vi "XYZ stage handler_MD.vi"   [LabVIEW 2012]
uses:
  <vilib>/Analysis/coordinate.llb/Euler Rotation Order.ctl
  GFG/GFGfpRefGet.vi
  GFG/GFGbooleanGet.vi
  GFG/GFGnumericGet.vi
  <vilib>/Analysis/coordinate.llb/3D Cartesian Coordinate Rotation (Euler) (Scalar).vi
  GFG/GFG library.lvlib
  <vilib>/Utility/VariantDataType/Type.ctl
  <vilib>/Utility/VariantDataType/VariantType.lvlib
  <vilib>/Analysis/NI_AALPro.lvlib
types:
  T1 = enum16{"none", "quit", "Press", "Long Press", "Long Press finished", "Short Press finished"}
  T2 = cluster{"WaveformChartRef":refnum<vi>, "DigitalRef":refnum<vi>, "ArrayRef":refnum<vi>, "TabControlRef":refnum<vi>, "EnumRef":refnum<vi>, "RingRef":refnum<vi>, "BooleanRef":refnum<vi>, "KnobRef":refnum<vi>, "SlideRef":refnum<vi>, "PathRef":refnum<vi>, "StringRef":refnum<vi>, "ComboBox":refnum<vi>, "WaveformGraphRef":refnum<vi>}
  T3 = cluster{"moveXabs":dbl, "moveYabs":dbl, "moveZabs":dbl}
  T4 = typedef "NI_AALPro.lvlib/Euler Rotation Order.ctl" = u16
  T5 = cluster{"Numeric":dbl, "Numeric":dbl, "Numeric":dbl}
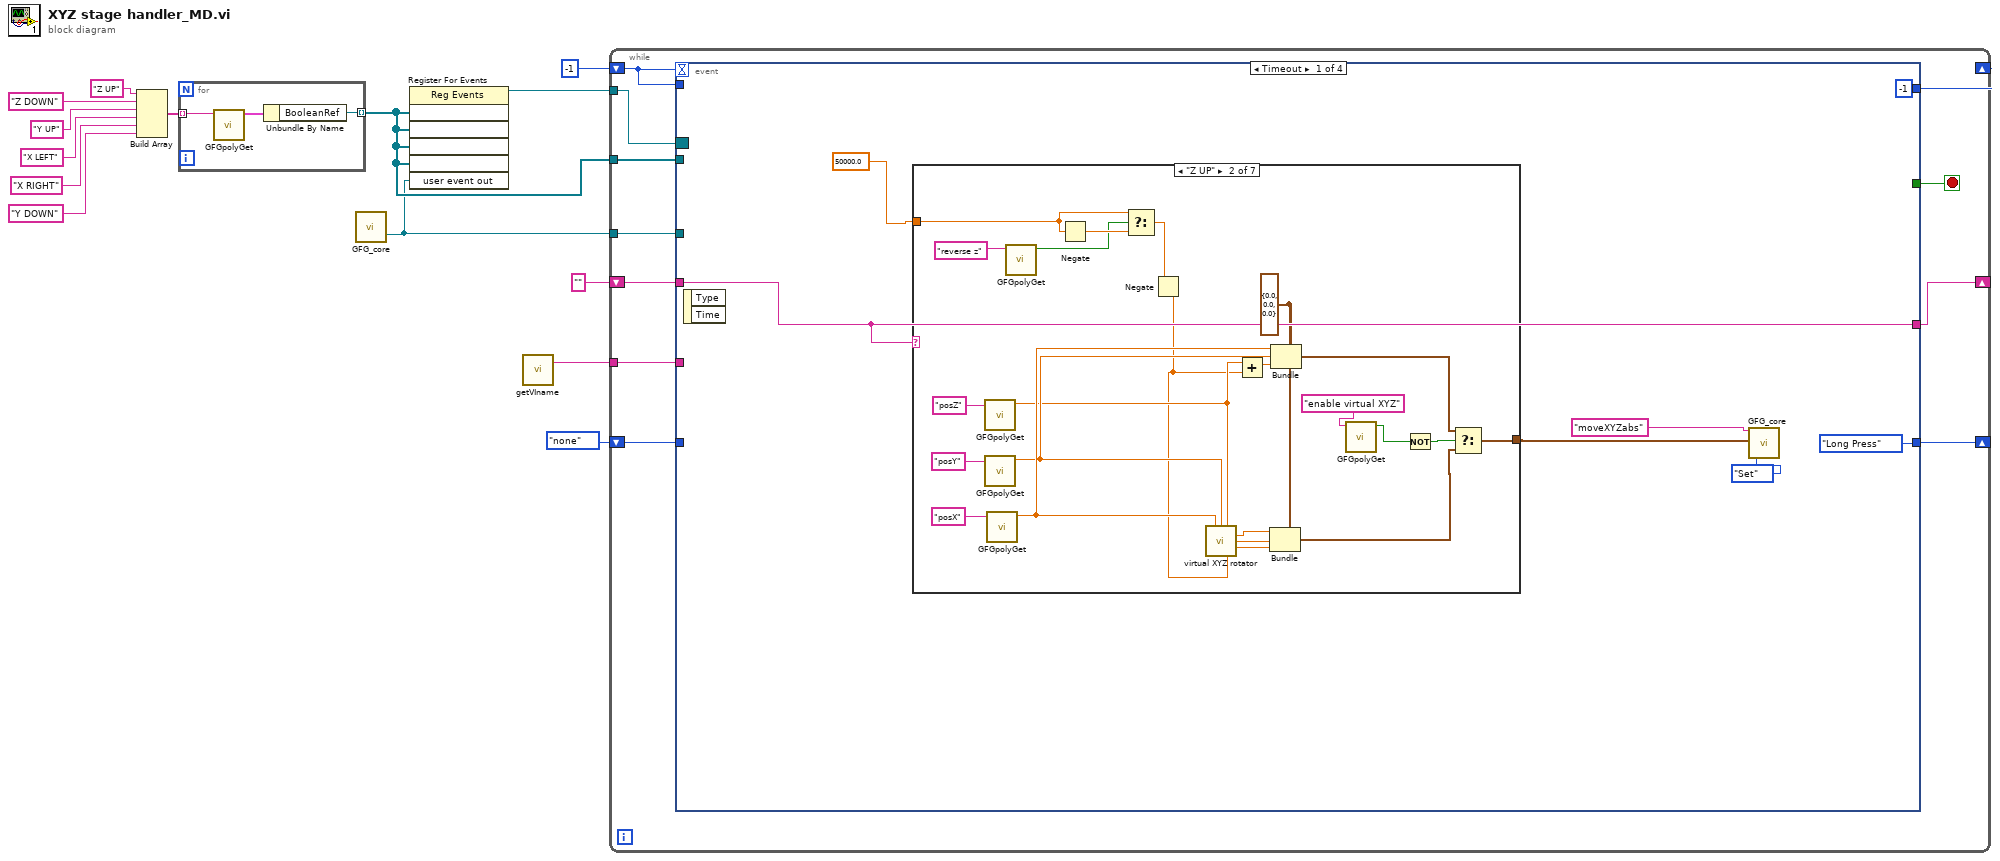
[diagram p0: block diagram]
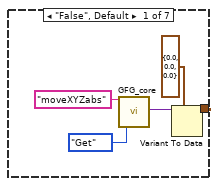
[diagram p2: hidden frame]
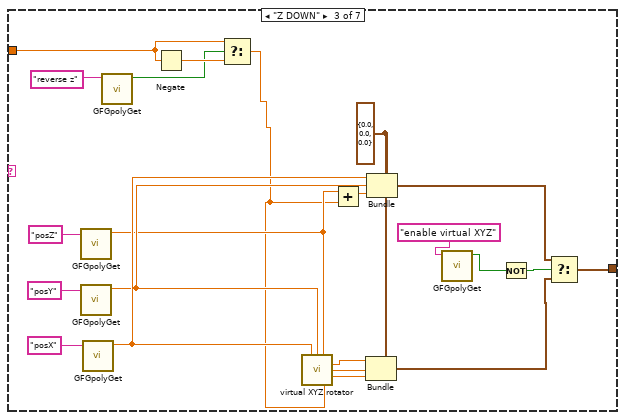
[diagram p3: hidden frame]
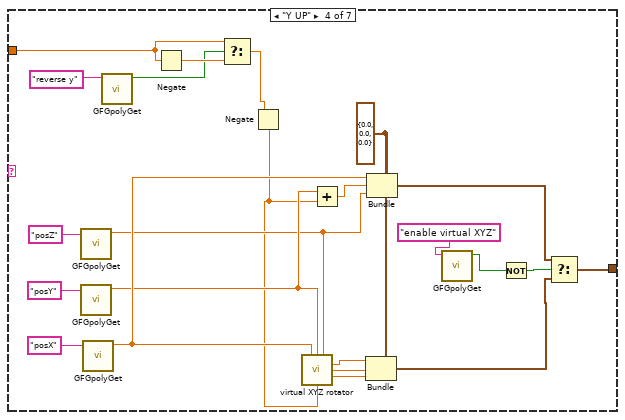
[diagram p4: hidden frame]
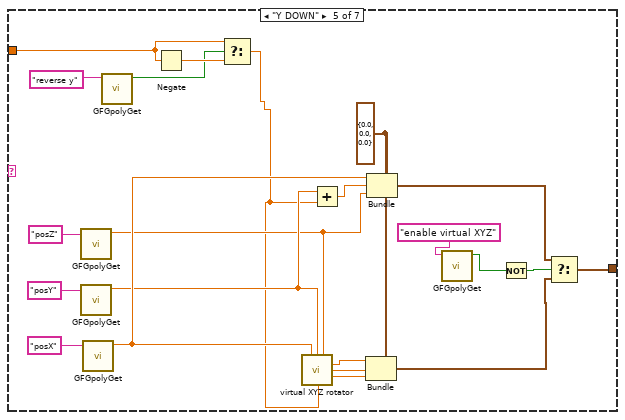
[diagram p5: hidden frame]
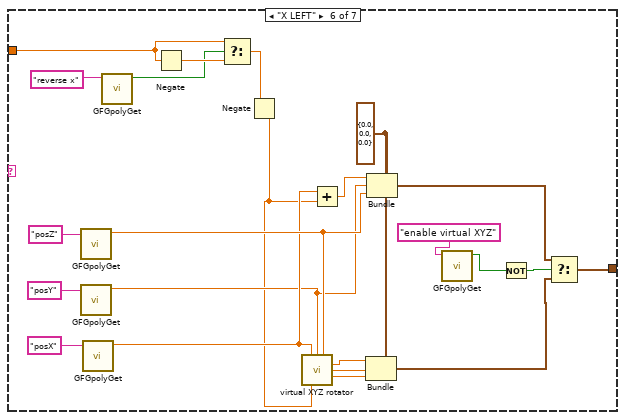
[diagram p6: hidden frame]
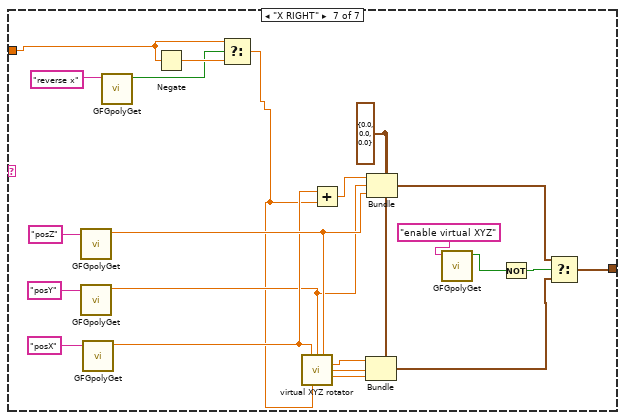
[diagram p7: hidden frame]
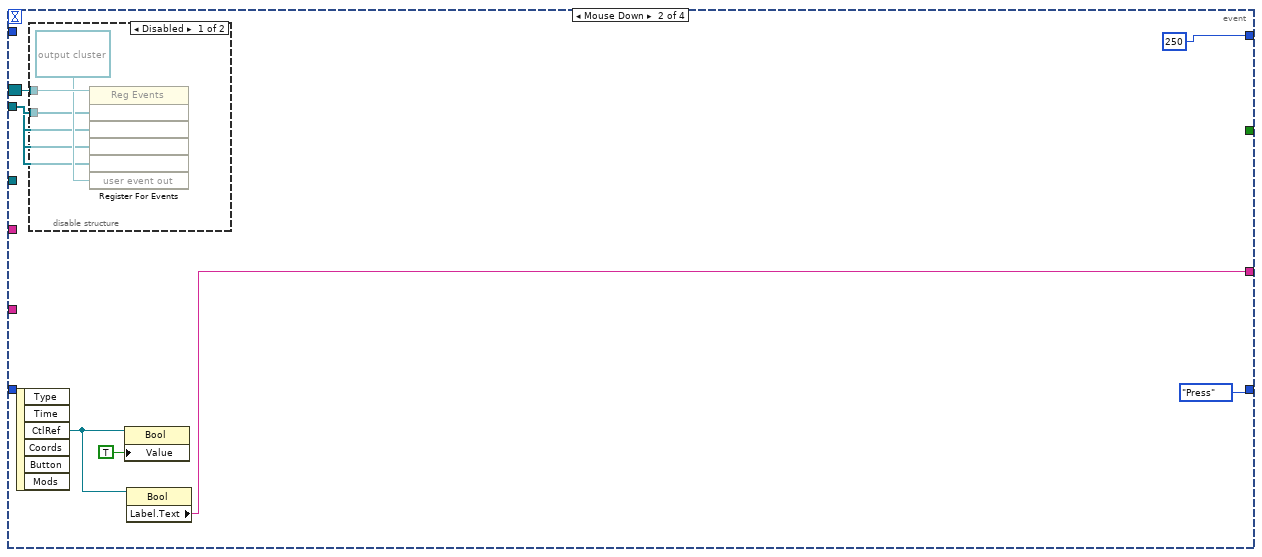
[diagram p8: hidden frame]
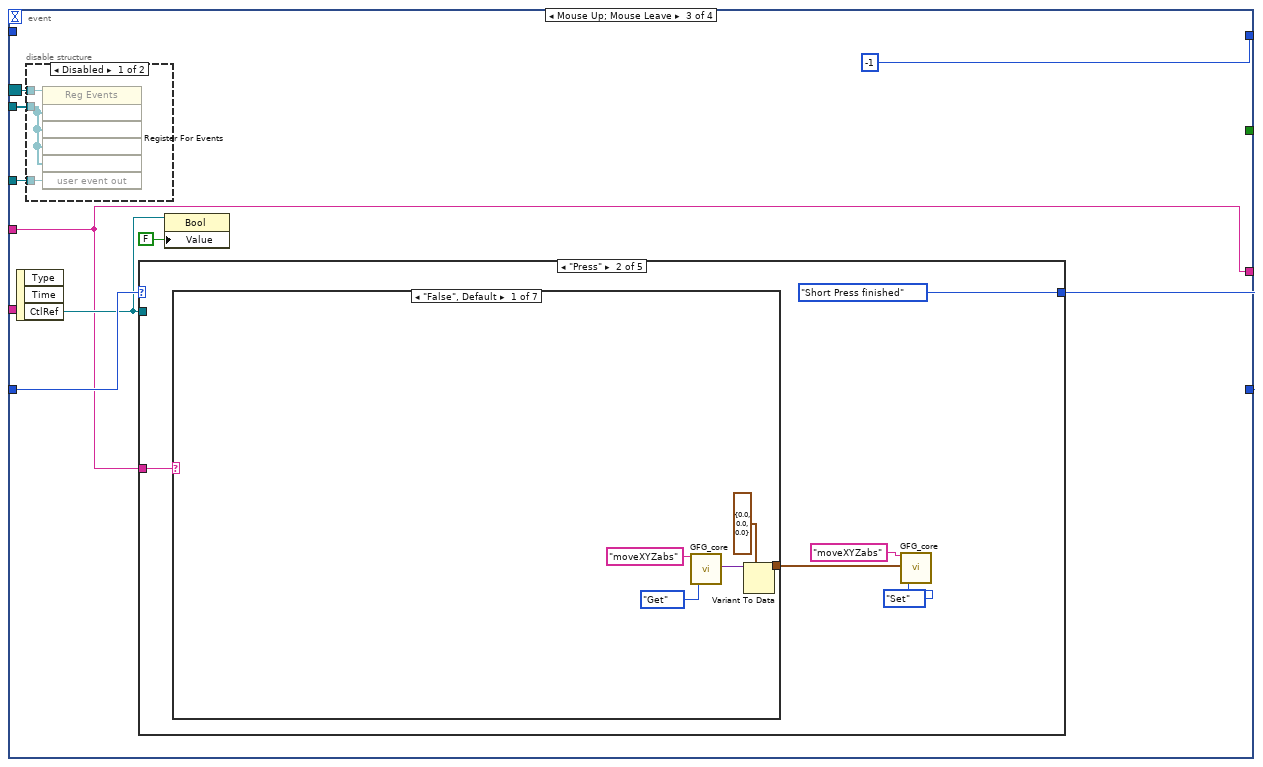
[diagram p10: hidden frame]
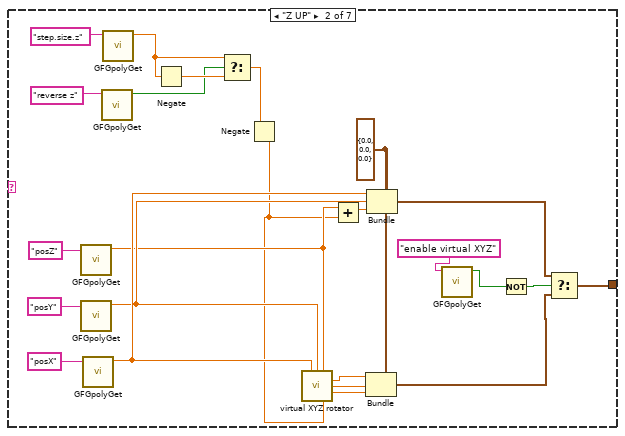
[diagram p13: hidden frame]
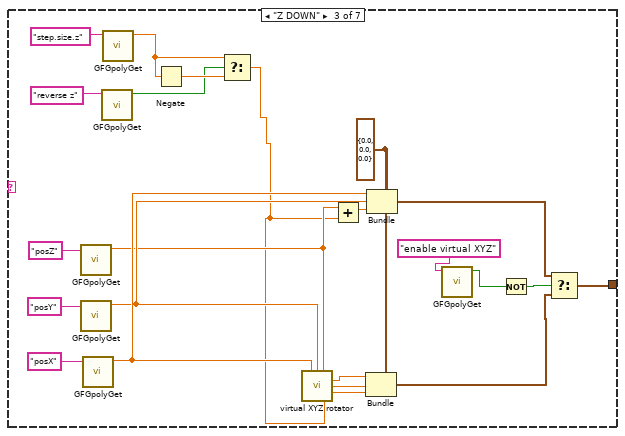
[diagram p14: hidden frame]
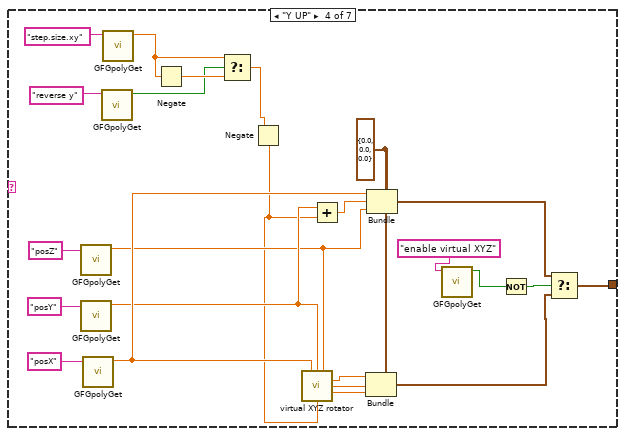
[diagram p15: hidden frame]
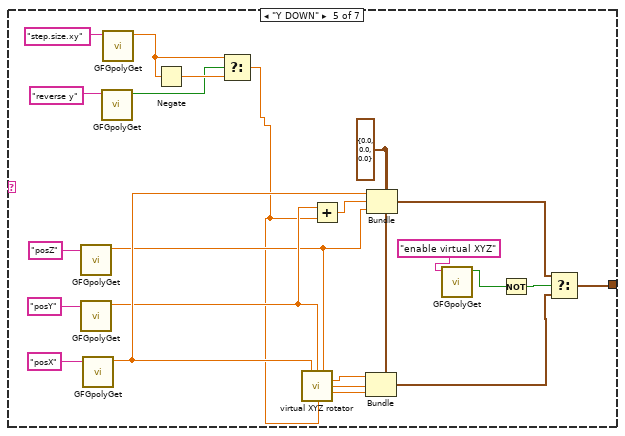
[diagram p16: hidden frame]
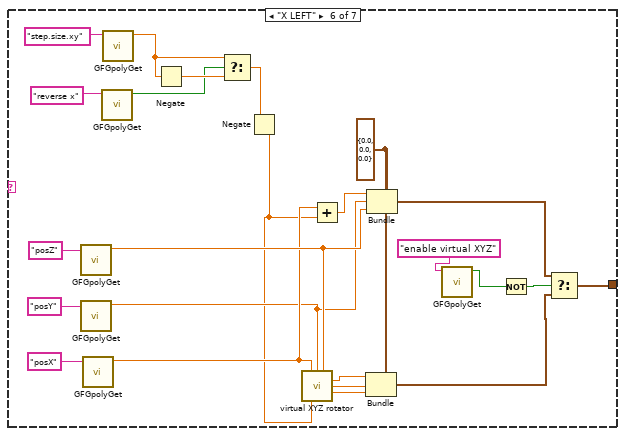
[diagram p17: hidden frame]
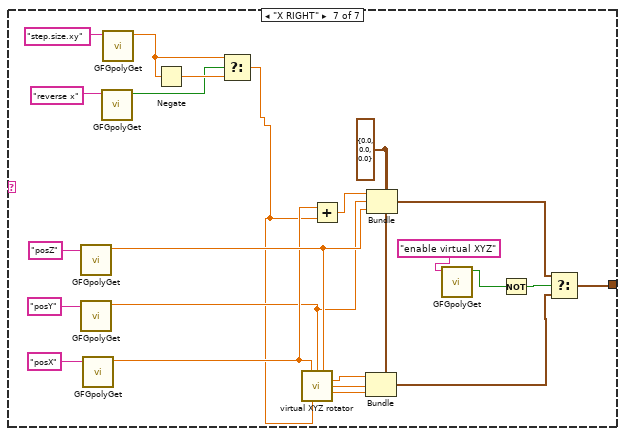
[diagram p18: hidden frame]
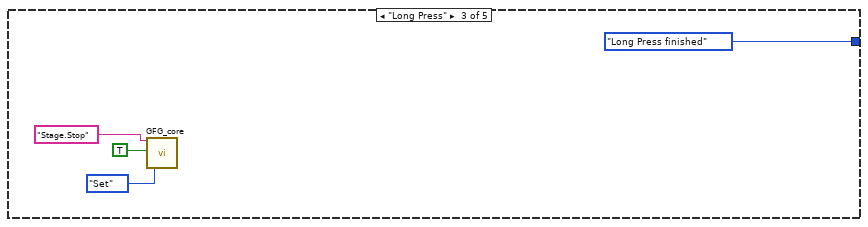
[diagram p19: hidden frame]
diagram:
  n1 = Build Array("Z UP" ("Variable Name in"), "Z DOWN" ("Variable Name in"), "Y UP" ("Variable Name in"), "X LEFT" ("Variable Name in"), "X RIGHT" ("Variable Name in"), "Y DOWN" ("Variable Name in")) -> (w11:string[])
  n2 = for {
    tunnel: w11 -> [w16] mode=indexing
    tunnel: [w15] -> w3 mode=indexing
    n3 = call-poly "GFGpolyGet.vi"("Variable Name in"=w16) -> ("output cluster"=w17:T2)  [unwired: 9 in, 1 out]
    n4 = Unbundle By Name(w17) -> ("BooleanRef"=w15:refnum<vi>)
  }
  n5 = call "GFG_core.vi"() -> ("user event out"=w2:refnum<user-event>)  [unwired: 13 in, 6 out]
  n6 = register-events(w3, w3, w3, w3, w2) -> (reference out=w4:refnum<event-registration>)  [unwired: 2 in, 1 out]
  n7 = call "getVIname.vi"() -> ("VI name"=w1:string)  [unwired: 19 in]
  n8 = while {
    shift-right: [w26] -> _
    shift-left: -1 -> [w27]
    shift-right: [w24] -> _
    shift-left: T1."none" ("Enum") -> [w25]
    shift-right: [w23] -> _
    shift-left: "" ("Label.Text") -> [w22]
    tunnel: w3 -> [w21]
    tunnel: w2 -> [w20]
    tunnel: w4 -> [w19]
    tunnel: w1 -> [w18]
    stop <- w28 stop-if-true
    n9 = event shown="[0] Timeout" {
      selector: w19 -> [_ w179 w188 _]
      dyn-events: _ -> [_ _ _ _]
      timeout: w27 -> [_ _ _ _]
      tunnel: [_ _ _ w361] -> w28
      tunnel: w27 -> [_ _ _ w359]
      tunnel: [-1 250 -1 w359] -> w26
      tunnel: w25 -> [_ _ w193 w360]
      tunnel: [T1."Long Press" ("Enum") T1."Press" ("Enum") w192 w360] -> w24
      tunnel: [w33 w180 w186 w356] -> w23
      tunnel: w22 -> [w33 _ w186 w356]
      tunnel: w21 -> [_ w176 w187 _]
      tunnel: w20 -> [_ _ w189 _]
      tunnel: w18 -> [_ _ _ w357]
      event Timeout {
        n10 = event-data() -> ()  [unwired: 1 in, 2 out]
        n11 = case shown="\"Z UP\"" w33 {
          tunnel: [w36 w46 w68 w94 w116 w140 w162] -> w29
          tunnel: 50000.0 ("-x") -> [_ w41 w64 w86 w109 w131 w154]
          frame "False", Default {
            n12 = call "GFG_core.vi"("Variable Name in"="moveXYZabs", "Action"=enum16{"Init", "Set", "Get"}."Get") -> ("Variant Out"=w38:variant)  [unwired: 11 in, 6 out]
            n13 = Variant To Data(type=T3 {"moveXabs"=0.0, "moveYabs"=0.0, "moveZabs"=0.0} ("output cluster"), Variant=w38) -> (data=w36:T3)  [unwired: 1 in, 1 out]
          }
          frame "Z UP" {
            w49 = T3 {"moveXabs"=0.0, "moveYabs"=0.0, "moveZabs"=0.0} ("output cluster")
            n14 = call-poly "GFGpolyGet.vi"("Variable Name in"="posZ") -> ("Numeric"=w53:dbl)  [unwired: 9 in, 1 out]
            n15 = call-poly "GFGpolyGet.vi"("Variable Name in"="posY") -> ("Numeric"=w54:dbl)  [unwired: 9 in, 1 out]
            n16 = call-poly "GFGpolyGet.vi"("Variable Name in"="posX") -> ("Numeric"=w55:dbl)  [unwired: 9 in, 1 out]
            n17 = call-poly "GFGpolyGet.vi"("Variable Name in"="reverse z") -> ("Boolean"=w61:bool)  [unwired: 10 in]
            n18 = Negate(x=w41) -> (-x=w62:dbl)
            n19 = Select(t=w41, s=w61, f=w62) -> (s? t:f=w43:dbl)
            n20 = Negate(x=w43) -> (-x=w42:dbl)
            n21 = call "virtual XYZ rotator.vi"("current pos X"=w55, "current pos Y"=w54, "current pos Z"=w53, "virtual Z relative"=w42) -> ("new pos X"=w52:dbl, "new pos Y"=w51:dbl, "new pos Z"=w50:dbl)  [unwired: 9 in]
            n22 = Add(x=w53, y=w42) -> (x+y=w57:dbl)
            n23 = Bundle(cluster=w49, "moveXabs"=w52, "moveYabs"=w51, "moveZabs"=w50) -> (w47:T3)
            n24 = Bundle(cluster=w49, "moveXabs"=w55, "moveYabs"=w54, "moveZabs"=w57) -> (w48:T3)
            n25 = call-poly "GFGpolyGet.vi"("Variable Name in"="enable virtual XYZ") -> ("Boolean"=w45:bool)  [unwired: 10 in]
            n26 = Not(x=w45) -> (.not. x?=w44:bool)
            n27 = Select(t=w48, s=w44, f=w47) -> (s? t:f=w46:T3)
          }
          frame "Z DOWN" {
            w71 = T3 {"moveXabs"=0.0, "moveYabs"=0.0, "moveZabs"=0.0} ("output cluster")
            n28 = call-poly "GFGpolyGet.vi"("Variable Name in"="posZ") -> ("Numeric"=w75:dbl)  [unwired: 9 in, 1 out]
            n29 = call-poly "GFGpolyGet.vi"("Variable Name in"="posY") -> ("Numeric"=w76:dbl)  [unwired: 9 in, 1 out]
            n30 = call-poly "GFGpolyGet.vi"("Variable Name in"="posX") -> ("Numeric"=w77:dbl)  [unwired: 9 in, 1 out]
            n31 = call-poly "GFGpolyGet.vi"("Variable Name in"="reverse z") -> ("Boolean"=w83:bool)  [unwired: 10 in]
            n32 = Negate(x=w64) -> (-x=w84:dbl)
            n33 = Select(t=w64, s=w83, f=w84) -> (s? t:f=w65:dbl)
            n34 = call "virtual XYZ rotator.vi"("current pos X"=w77, "current pos Y"=w76, "current pos Z"=w75, "virtual Z relative"=w65) -> ("new pos X"=w74:dbl, "new pos Y"=w73:dbl, "new pos Z"=w72:dbl)  [unwired: 9 in]
            n35 = Add(x=w75, y=w65) -> (x+y=w79:dbl)
            n36 = Bundle(cluster=w71, "moveXabs"=w74, "moveYabs"=w73, "moveZabs"=w72) -> (w69:T3)
            n37 = Bundle(cluster=w71, "moveXabs"=w77, "moveYabs"=w76, "moveZabs"=w79) -> (w70:T3)
            n38 = call-poly "GFGpolyGet.vi"("Variable Name in"="enable virtual XYZ") -> ("Boolean"=w67:bool)  [unwired: 10 in]
            n39 = Not(x=w67) -> (.not. x?=w66:bool)
            n40 = Select(t=w70, s=w66, f=w69) -> (s? t:f=w68:T3)
          }
          frame "Y UP" {
            w97 = T3 {"moveXabs"=0.0, "moveYabs"=0.0, "moveZabs"=0.0} ("output cluster")
            n41 = call-poly "GFGpolyGet.vi"("Variable Name in"="posZ") -> ("Numeric"=w88:dbl)  [unwired: 9 in, 1 out]
            n42 = call-poly "GFGpolyGet.vi"("Variable Name in"="posY") -> ("Numeric"=w90:dbl)  [unwired: 9 in, 1 out]
            n43 = call-poly "GFGpolyGet.vi"("Variable Name in"="posX") -> ("Numeric"=w101:dbl)  [unwired: 9 in, 1 out]
            n44 = call-poly "GFGpolyGet.vi"("Variable Name in"="reverse y") -> ("Boolean"=w106:bool)  [unwired: 10 in]
            n45 = Negate(x=w86) -> (-x=w107:dbl)
            n46 = Select(t=w86, s=w106, f=w107) -> (s? t:f=w91:dbl)
            n47 = Negate(x=w91) -> (-x=w87:dbl)
            n48 = call "virtual XYZ rotator.vi"("current pos X"=w101, "current pos Y"=w90, "current pos Z"=w88, "virtual Y relative"=w87) -> ("new pos X"=w100:dbl, "new pos Y"=w99:dbl, "new pos Z"=w98:dbl)  [unwired: 9 in]
            n49 = Add(x=w90, y=w87) -> (x+y=w89:dbl)
            n50 = Bundle(cluster=w97, "moveXabs"=w100, "moveYabs"=w99, "moveZabs"=w98) -> (w95:T3)
            n51 = Bundle(cluster=w97, "moveXabs"=w101, "moveYabs"=w89, "moveZabs"=w88) -> (w96:T3)
            n52 = call-poly "GFGpolyGet.vi"("Variable Name in"="enable virtual XYZ") -> ("Boolean"=w93:bool)  [unwired: 10 in]
            n53 = Not(x=w93) -> (.not. x?=w92:bool)
            n54 = Select(t=w96, s=w92, f=w95) -> (s? t:f=w94:T3)
          }
          frame "Y DOWN" {
            w119 = T3 {"moveXabs"=0.0, "moveYabs"=0.0, "moveZabs"=0.0} ("output cluster")
            n55 = call-poly "GFGpolyGet.vi"("Variable Name in"="posZ") -> ("Numeric"=w111:dbl)  [unwired: 9 in, 1 out]
            n56 = call-poly "GFGpolyGet.vi"("Variable Name in"="posY") -> ("Numeric"=w113:dbl)  [unwired: 9 in, 1 out]
            n57 = call-poly "GFGpolyGet.vi"("Variable Name in"="posX") -> ("Numeric"=w123:dbl)  [unwired: 9 in, 1 out]
            n58 = call-poly "GFGpolyGet.vi"("Variable Name in"="reverse y") -> ("Boolean"=w128:bool)  [unwired: 10 in]
            n59 = Negate(x=w109) -> (-x=w129:dbl)
            n60 = Select(t=w109, s=w128, f=w129) -> (s? t:f=w110:dbl)
            n61 = call "virtual XYZ rotator.vi"("current pos X"=w123, "current pos Y"=w113, "current pos Z"=w111, "virtual Y relative"=w110) -> ("new pos X"=w122:dbl, "new pos Y"=w121:dbl, "new pos Z"=w120:dbl)  [unwired: 9 in]
            n62 = Add(x=w113, y=w110) -> (x+y=w112:dbl)
            n63 = Bundle(cluster=w119, "moveXabs"=w122, "moveYabs"=w121, "moveZabs"=w120) -> (w117:T3)
            n64 = Bundle(cluster=w119, "moveXabs"=w123, "moveYabs"=w112, "moveZabs"=w111) -> (w118:T3)
            n65 = call-poly "GFGpolyGet.vi"("Variable Name in"="enable virtual XYZ") -> ("Boolean"=w115:bool)  [unwired: 10 in]
            n66 = Not(x=w115) -> (.not. x?=w114:bool)
            n67 = Select(t=w118, s=w114, f=w117) -> (s? t:f=w116:T3)
          }
          frame "X LEFT" {
            w143 = T3 {"moveXabs"=0.0, "moveYabs"=0.0, "moveZabs"=0.0} ("output cluster")
            n68 = call-poly "GFGpolyGet.vi"("Variable Name in"="posZ") -> ("Numeric"=w137:dbl)  [unwired: 9 in, 1 out]
            n69 = call-poly "GFGpolyGet.vi"("Variable Name in"="posY") -> ("Numeric"=w134:dbl)  [unwired: 9 in, 1 out]
            n70 = call-poly "GFGpolyGet.vi"("Variable Name in"="posX") -> ("Numeric"=w136:dbl)  [unwired: 9 in, 1 out]
            n71 = call-poly "GFGpolyGet.vi"("Variable Name in"="reverse x") -> ("Boolean"=w151:bool)  [unwired: 10 in]
            n72 = Negate(x=w131) -> (-x=w152:dbl)
            n73 = Select(t=w131, s=w151, f=w152) -> (s? t:f=w133:dbl)
            n74 = Negate(x=w133) -> (-x=w132:dbl)
            n75 = call "virtual XYZ rotator.vi"("current pos X"=w136, "current pos Y"=w134, "current pos Z"=w137, "virtual X relative"=w132) -> ("new pos X"=w146:dbl, "new pos Y"=w145:dbl, "new pos Z"=w144:dbl)  [unwired: 9 in]
            n76 = Add(x=w136, y=w132) -> (x+y=w135:dbl)
            n77 = Bundle(cluster=w143, "moveXabs"=w146, "moveYabs"=w145, "moveZabs"=w144) -> (w141:T3)
            n78 = Bundle(cluster=w143, "moveXabs"=w135, "moveYabs"=w134, "moveZabs"=w137) -> (w142:T3)
            n79 = call-poly "GFGpolyGet.vi"("Variable Name in"="enable virtual XYZ") -> ("Boolean"=w139:bool)  [unwired: 10 in]
            n80 = Not(x=w139) -> (.not. x?=w138:bool)
            n81 = Select(t=w142, s=w138, f=w141) -> (s? t:f=w140:T3)
          }
          frame "X RIGHT" {
            w165 = T3 {"moveXabs"=0.0, "moveYabs"=0.0, "moveZabs"=0.0} ("output cluster")
            n82 = call-poly "GFGpolyGet.vi"("Variable Name in"="posZ") -> ("Numeric"=w159:dbl)  [unwired: 9 in, 1 out]
            n83 = call-poly "GFGpolyGet.vi"("Variable Name in"="posY") -> ("Numeric"=w156:dbl)  [unwired: 9 in, 1 out]
            n84 = call-poly "GFGpolyGet.vi"("Variable Name in"="posX") -> ("Numeric"=w158:dbl)  [unwired: 9 in, 1 out]
            n85 = call-poly "GFGpolyGet.vi"("Variable Name in"="reverse x") -> ("Boolean"=w173:bool)  [unwired: 10 in]
            n86 = Negate(x=w154) -> (-x=w174:dbl)
            n87 = Select(t=w154, s=w173, f=w174) -> (s? t:f=w155:dbl)
            n88 = call "virtual XYZ rotator.vi"("current pos X"=w158, "current pos Y"=w156, "current pos Z"=w159, "virtual X relative"=w155) -> ("new pos X"=w168:dbl, "new pos Y"=w167:dbl, "new pos Z"=w166:dbl)  [unwired: 9 in]
            n89 = Add(x=w158, y=w155) -> (x+y=w157:dbl)
            n90 = Bundle(cluster=w165, "moveXabs"=w168, "moveYabs"=w167, "moveZabs"=w166) -> (w163:T3)
            n91 = Bundle(cluster=w165, "moveXabs"=w157, "moveYabs"=w156, "moveZabs"=w159) -> (w164:T3)
            n92 = call-poly "GFGpolyGet.vi"("Variable Name in"="enable virtual XYZ") -> ("Boolean"=w161:bool)  [unwired: 10 in]
            n93 = Not(x=w161) -> (.not. x?=w160:bool)
            n94 = Select(t=w164, s=w160, f=w163) -> (s? t:f=w162:T3)
          }
        }
        n95 = call "GFG_core.vi"("Variable Name in"="moveXYZabs", "Variant in"=w29, "Action"=enum16{"Init", "Set", "Get"}."Set") -> ()  [unwired: 10 in, 7 out]
      }
      event Mouse Down {
        n96 = event-data() -> ("CtlRef"=w178:refnum<vi>)  [unwired: 1 in, 5 out]
        n97 = disable-structure shown="Disabled" {
          disable-tunnel: w179 -> [w185 _]
          disable-tunnel: w176 -> [w183 _]
          frame Disabled {
            n98 = register-events(reference=w185, w183, w183, w183, w183, refnum<user-event> refnum ("event source")) -> ()  [unwired: 1 in, 2 out]
          }
          frame Enabled {
          }
        }
        n99 = property class="Bool"(reference=w178, "Value"=TRUE) -> ()  [unwired: 1 in, 2 out]
        n100 = property class="Bool"(reference=w178) -> ("Label.Text"=w180:string)  [unwired: 1 in, 2 out]
      }
      event Mouse Up; Mouse Leave {
        n101 = event-data() -> ("CtlRef"=w191:refnum<vi>)  [unwired: 1 in, 2 out]
        n102 = disable-structure shown="Disabled" {
          disable-tunnel: w189 -> [w197 _]
          disable-tunnel: w188 -> [w196 _]
          disable-tunnel: w187 -> [w195 _]
          frame Disabled {
            n103 = register-events(reference=w196, w195, w195, w195, w195, w197) -> ()  [unwired: 1 in, 2 out]
          }
          frame Enabled {
          }
        }
        n104 = case shown="\"Press\"" w193 {
          selector: w193 -> [w198 _ _ w354 w355]
          tunnel: [w198 T1."Short Press finished" ("Enum") T1."Long Press finished" ("Enum") w354 w355] -> w192
          tunnel: w191 -> [_ _ _ _ _]
          tunnel: w186 -> [_ w202 _ _ _]
          frame "none", Default {
          }
          frame "Press" {
            n105 = case shown="\"False\", Default" w202 {
              tunnel: [w204 w213 w236 w263 w286 w311 w334] -> w199
              frame "False", Default {
                n106 = call "GFG_core.vi"("Variable Name in"="moveXYZabs", "Action"=enum16{"Init", "Set", "Get"}."Get") -> ("Variant Out"=w206:variant)  [unwired: 11 in, 6 out]
                n107 = Variant To Data(type=T3 {"moveXabs"=0.0, "moveYabs"=0.0, "moveZabs"=0.0} ("output cluster"), Variant=w206) -> (data=w204:T3)  [unwired: 1 in, 1 out]
              }
              frame "Z UP" {
                w216 = T3 {"moveXabs"=0.0, "moveYabs"=0.0, "moveZabs"=0.0} ("output cluster")
                n108 = call-poly "GFGpolyGet.vi"("Variable Name in"="posZ") -> ("Numeric"=w220:dbl)  [unwired: 9 in, 1 out]
                n109 = call-poly "GFGpolyGet.vi"("Variable Name in"="posY") -> ("Numeric"=w221:dbl)  [unwired: 9 in, 1 out]
                n110 = call-poly "GFGpolyGet.vi"("Variable Name in"="posX") -> ("Numeric"=w222:dbl)  [unwired: 9 in, 1 out]
                n111 = call-poly "GFGpolyGet.vi"("Variable Name in"="reverse z") -> ("Boolean"=w228:bool)  [unwired: 10 in]
                n112 = call-poly "GFGpolyGet.vi"("Variable Name in"="step.size.z") -> ("Numeric"=w229:dbl)  [unwired: 9 in, 1 out]
                n113 = Negate(x=w229) -> (-x=w230:dbl)
                n114 = Select(t=w229, s=w228, f=w230) -> (s? t:f=w210:dbl)
                n115 = Negate(x=w210) -> (-x=w209:dbl)
                n116 = call "virtual XYZ rotator.vi"("current pos X"=w222, "current pos Y"=w221, "current pos Z"=w220, "virtual Z relative"=w209) -> ("new pos X"=w219:dbl, "new pos Y"=w218:dbl, "new pos Z"=w217:dbl)  [unwired: 9 in]
                n117 = Add(x=w220, y=w209) -> (x+y=w224:dbl)
                n118 = Bundle(cluster=w216, "moveXabs"=w219, "moveYabs"=w218, "moveZabs"=w217) -> (w214:T3)
                n119 = Bundle(cluster=w216, "moveXabs"=w222, "moveYabs"=w221, "moveZabs"=w224) -> (w215:T3)
                n120 = call-poly "GFGpolyGet.vi"("Variable Name in"="enable virtual XYZ") -> ("Boolean"=w212:bool)  [unwired: 10 in]
                n121 = Not(x=w212) -> (.not. x?=w211:bool)
                n122 = Select(t=w215, s=w211, f=w214) -> (s? t:f=w213:T3)
              }
              frame "Z DOWN" {
                w239 = T3 {"moveXabs"=0.0, "moveYabs"=0.0, "moveZabs"=0.0} ("output cluster")
                n123 = call-poly "GFGpolyGet.vi"("Variable Name in"="posZ") -> ("Numeric"=w243:dbl)  [unwired: 9 in, 1 out]
                n124 = call-poly "GFGpolyGet.vi"("Variable Name in"="posY") -> ("Numeric"=w244:dbl)  [unwired: 9 in, 1 out]
                n125 = call-poly "GFGpolyGet.vi"("Variable Name in"="posX") -> ("Numeric"=w245:dbl)  [unwired: 9 in, 1 out]
                n126 = call-poly "GFGpolyGet.vi"("Variable Name in"="reverse z") -> ("Boolean"=w251:bool)  [unwired: 10 in]
                n127 = call-poly "GFGpolyGet.vi"("Variable Name in"="step.size.z") -> ("Numeric"=w252:dbl)  [unwired: 9 in, 1 out]
                n128 = Negate(x=w252) -> (-x=w253:dbl)
                n129 = Select(t=w252, s=w251, f=w253) -> (s? t:f=w233:dbl)
                n130 = call "virtual XYZ rotator.vi"("current pos X"=w245, "current pos Y"=w244, "current pos Z"=w243, "virtual Z relative"=w233) -> ("new pos X"=w242:dbl, "new pos Y"=w241:dbl, "new pos Z"=w240:dbl)  [unwired: 9 in]
                n131 = Add(x=w243, y=w233) -> (x+y=w247:dbl)
                n132 = Bundle(cluster=w239, "moveXabs"=w242, "moveYabs"=w241, "moveZabs"=w240) -> (w237:T3)
                n133 = Bundle(cluster=w239, "moveXabs"=w245, "moveYabs"=w244, "moveZabs"=w247) -> (w238:T3)
                n134 = call-poly "GFGpolyGet.vi"("Variable Name in"="enable virtual XYZ") -> ("Boolean"=w235:bool)  [unwired: 10 in]
                n135 = Not(x=w235) -> (.not. x?=w234:bool)
                n136 = Select(t=w238, s=w234, f=w237) -> (s? t:f=w236:T3)
              }
              frame "Y UP" {
                w266 = T3 {"moveXabs"=0.0, "moveYabs"=0.0, "moveZabs"=0.0} ("output cluster")
                n137 = call-poly "GFGpolyGet.vi"("Variable Name in"="posZ") -> ("Numeric"=w257:dbl)  [unwired: 9 in, 1 out]
                n138 = call-poly "GFGpolyGet.vi"("Variable Name in"="posY") -> ("Numeric"=w259:dbl)  [unwired: 9 in, 1 out]
                n139 = call-poly "GFGpolyGet.vi"("Variable Name in"="posX") -> ("Numeric"=w270:dbl)  [unwired: 9 in, 1 out]
                n140 = call-poly "GFGpolyGet.vi"("Variable Name in"="reverse y") -> ("Boolean"=w275:bool)  [unwired: 10 in]
                n141 = call-poly "GFGpolyGet.vi"("Variable Name in"="step.size.xy") -> ("Numeric"=w276:dbl)  [unwired: 9 in, 1 out]
                n142 = Negate(x=w276) -> (-x=w277:dbl)
                n143 = Select(t=w276, s=w275, f=w277) -> (s? t:f=w260:dbl)
                n144 = Negate(x=w260) -> (-x=w256:dbl)
                n145 = call "virtual XYZ rotator.vi"("current pos X"=w270, "current pos Y"=w259, "current pos Z"=w257, "virtual Y relative"=w256) -> ("new pos X"=w269:dbl, "new pos Y"=w268:dbl, "new pos Z"=w267:dbl)  [unwired: 9 in]
                n146 = Add(x=w259, y=w256) -> (x+y=w258:dbl)
                n147 = Bundle(cluster=w266, "moveXabs"=w269, "moveYabs"=w268, "moveZabs"=w267) -> (w264:T3)
                n148 = Bundle(cluster=w266, "moveXabs"=w270, "moveYabs"=w258, "moveZabs"=w257) -> (w265:T3)
                n149 = call-poly "GFGpolyGet.vi"("Variable Name in"="enable virtual XYZ") -> ("Boolean"=w262:bool)  [unwired: 10 in]
                n150 = Not(x=w262) -> (.not. x?=w261:bool)
                n151 = Select(t=w265, s=w261, f=w264) -> (s? t:f=w263:T3)
              }
              frame "Y DOWN" {
                w289 = T3 {"moveXabs"=0.0, "moveYabs"=0.0, "moveZabs"=0.0} ("output cluster")
                n152 = call-poly "GFGpolyGet.vi"("Variable Name in"="posZ") -> ("Numeric"=w281:dbl)  [unwired: 9 in, 1 out]
                n153 = call-poly "GFGpolyGet.vi"("Variable Name in"="posY") -> ("Numeric"=w283:dbl)  [unwired: 9 in, 1 out]
                n154 = call-poly "GFGpolyGet.vi"("Variable Name in"="posX") -> ("Numeric"=w293:dbl)  [unwired: 9 in, 1 out]
                n155 = call-poly "GFGpolyGet.vi"("Variable Name in"="reverse y") -> ("Boolean"=w298:bool)  [unwired: 10 in]
                n156 = call-poly "GFGpolyGet.vi"("Variable Name in"="step.size.xy") -> ("Numeric"=w299:dbl)  [unwired: 9 in, 1 out]
                n157 = Negate(x=w299) -> (-x=w300:dbl)
                n158 = Select(t=w299, s=w298, f=w300) -> (s? t:f=w280:dbl)
                n159 = call "virtual XYZ rotator.vi"("current pos X"=w293, "current pos Y"=w283, "current pos Z"=w281, "virtual Y relative"=w280) -> ("new pos X"=w292:dbl, "new pos Y"=w291:dbl, "new pos Z"=w290:dbl)  [unwired: 9 in]
                n160 = Add(x=w283, y=w280) -> (x+y=w282:dbl)
                n161 = Bundle(cluster=w289, "moveXabs"=w292, "moveYabs"=w291, "moveZabs"=w290) -> (w287:T3)
                n162 = Bundle(cluster=w289, "moveXabs"=w293, "moveYabs"=w282, "moveZabs"=w281) -> (w288:T3)
                n163 = call-poly "GFGpolyGet.vi"("Variable Name in"="enable virtual XYZ") -> ("Boolean"=w285:bool)  [unwired: 10 in]
                n164 = Not(x=w285) -> (.not. x?=w284:bool)
                n165 = Select(t=w288, s=w284, f=w287) -> (s? t:f=w286:T3)
              }
              frame "X LEFT" {
                w314 = T3 {"moveXabs"=0.0, "moveYabs"=0.0, "moveZabs"=0.0} ("output cluster")
                n166 = call-poly "GFGpolyGet.vi"("Variable Name in"="posZ") -> ("Numeric"=w308:dbl)  [unwired: 9 in, 1 out]
                n167 = call-poly "GFGpolyGet.vi"("Variable Name in"="posY") -> ("Numeric"=w305:dbl)  [unwired: 9 in, 1 out]
                n168 = call-poly "GFGpolyGet.vi"("Variable Name in"="posX") -> ("Numeric"=w307:dbl)  [unwired: 9 in, 1 out]
                n169 = call-poly "GFGpolyGet.vi"("Variable Name in"="reverse x") -> ("Boolean"=w322:bool)  [unwired: 10 in]
                n170 = call-poly "GFGpolyGet.vi"("Variable Name in"="step.size.xy") -> ("Numeric"=w323:dbl)  [unwired: 9 in, 1 out]
                n171 = Negate(x=w323) -> (-x=w324:dbl)
                n172 = Select(t=w323, s=w322, f=w324) -> (s? t:f=w304:dbl)
                n173 = Negate(x=w304) -> (-x=w303:dbl)
                n174 = call "virtual XYZ rotator.vi"("current pos X"=w307, "current pos Y"=w305, "current pos Z"=w308, "virtual X relative"=w303) -> ("new pos X"=w317:dbl, "new pos Y"=w316:dbl, "new pos Z"=w315:dbl)  [unwired: 9 in]
                n175 = Add(x=w307, y=w303) -> (x+y=w306:dbl)
                n176 = Bundle(cluster=w314, "moveXabs"=w317, "moveYabs"=w316, "moveZabs"=w315) -> (w312:T3)
                n177 = Bundle(cluster=w314, "moveXabs"=w306, "moveYabs"=w305, "moveZabs"=w308) -> (w313:T3)
                n178 = call-poly "GFGpolyGet.vi"("Variable Name in"="enable virtual XYZ") -> ("Boolean"=w310:bool)  [unwired: 10 in]
                n179 = Not(x=w310) -> (.not. x?=w309:bool)
                n180 = Select(t=w313, s=w309, f=w312) -> (s? t:f=w311:T3)
              }
              frame "X RIGHT" {
                w337 = T3 {"moveXabs"=0.0, "moveYabs"=0.0, "moveZabs"=0.0} ("output cluster")
                n181 = call-poly "GFGpolyGet.vi"("Variable Name in"="posZ") -> ("Numeric"=w331:dbl)  [unwired: 9 in, 1 out]
                n182 = call-poly "GFGpolyGet.vi"("Variable Name in"="posY") -> ("Numeric"=w328:dbl)  [unwired: 9 in, 1 out]
                n183 = call-poly "GFGpolyGet.vi"("Variable Name in"="posX") -> ("Numeric"=w330:dbl)  [unwired: 9 in, 1 out]
                n184 = call-poly "GFGpolyGet.vi"("Variable Name in"="reverse x") -> ("Boolean"=w345:bool)  [unwired: 10 in]
                n185 = call-poly "GFGpolyGet.vi"("Variable Name in"="step.size.xy") -> ("Numeric"=w346:dbl)  [unwired: 9 in, 1 out]
                n186 = Negate(x=w346) -> (-x=w347:dbl)
                n187 = Select(t=w346, s=w345, f=w347) -> (s? t:f=w327:dbl)
                n188 = call "virtual XYZ rotator.vi"("current pos X"=w330, "current pos Y"=w328, "current pos Z"=w331, "virtual X relative"=w327) -> ("new pos X"=w340:dbl, "new pos Y"=w339:dbl, "new pos Z"=w338:dbl)  [unwired: 9 in]
                n189 = Add(x=w330, y=w327) -> (x+y=w329:dbl)
                n190 = Bundle(cluster=w337, "moveXabs"=w340, "moveYabs"=w339, "moveZabs"=w338) -> (w335:T3)
                n191 = Bundle(cluster=w337, "moveXabs"=w329, "moveYabs"=w328, "moveZabs"=w331) -> (w336:T3)
                n192 = call-poly "GFGpolyGet.vi"("Variable Name in"="enable virtual XYZ") -> ("Boolean"=w333:bool)  [unwired: 10 in]
                n193 = Not(x=w333) -> (.not. x?=w332:bool)
                n194 = Select(t=w336, s=w332, f=w335) -> (s? t:f=w334:T3)
              }
            }
            n195 = call "GFG_core.vi"("Variable Name in"="moveXYZabs", "Variant in"=w199, "Action"=enum16{"Init", "Set", "Get"}."Set") -> ()  [unwired: 10 in, 7 out]
          }
          frame "Long Press" {
            n196 = call "GFG_core.vi"("Variable Name in"="Stage.Stop", "Variant in"=TRUE, "Action"=enum16{"Init", "Set", "Get"}."Set") -> ()  [unwired: 10 in, 7 out]
          }
          frame "Long Press finished" {
          }
          frame "Short Press finished" {
          }
        }
        n197 = property class="Bool"(reference=w191, "Value"=FALSE) -> ()  [unwired: 1 in, 2 out]
      }
      event User Event {
        n198 = event-data() -> ("Source VI"=w358:string, "Variable Name"=w362:string, "Variant"=w363:variant)  [unwired: 1 in, 4 out]
        n199 = case shown="\"setX\", \"setY\", \"setZ\"" w362 {
          selector: w362 -> [_ w365 w442 _ w458]
          tunnel: [_ _ _ w452 _] -> w361
          tunnel: w363 -> [_ w364 w441 w454 _]
          tunnel: w358 -> [_ w368 _ _ _]
          tunnel: w357 -> [_ w367 _ _ _]
          frame "False", Default {
          }
          frame "setX", "setY", "setZ" {
            n200 = Not Equal?(x=w367, y=w368) -> (x != y?=w366:bool)
            n201 = case shown="True" w366 {
              tunnel: w365 -> [_ w386]
              tunnel: w364 -> [_ w385]
              frame False {
              }
              frame True {
                w375 = 0.0 ("current pos X")
                w380 = T3 {"moveXabs"=0.0, "moveYabs"=0.0, "moveZabs"=0.0} ("output cluster")
                n202 = call-poly "GFGpolyGet.vi"("Variable Name in"="setX") -> ("Numeric"=w391:dbl)  [unwired: 9 in, 1 out]
                n203 = call-poly "GFGpolyGet.vi"("Variable Name in"="setY") -> ("Numeric"=w390:dbl)  [unwired: 9 in, 1 out]
                n204 = call-poly "GFGpolyGet.vi"("Variable Name in"="setZ") -> ("Numeric"=w392:dbl)  [unwired: 9 in, 1 out]
                n205 = case shown="\"setZ\"" w386 {
                  tunnel: w390 -> [w394 w399 w402 w408]
                  tunnel: w391 -> [w395 w398 w403 w409]
                  tunnel: w392 -> [w393 w396 w404 w407]
                  tunnel: w385 -> [_ w400 w405 w410]
                  tunnel: [w394 w399 w401 w408] -> w370
                  tunnel: [w395 w397 w403 w409] -> w371
                  tunnel: [w393 w396 w404 w406] -> w369
                  frame "False", Default {
                  }
                  frame "setX" {
                    n206 = Variant To Data(type=w398, Variant=w400) -> (data=w397:dbl)  [unwired: 1 in, 1 out]
                  }
                  frame "setY" {
                    n207 = Variant To Data(type=w402, Variant=w405) -> (data=w401:dbl)  [unwired: 1 in, 1 out]
                  }
                  frame "setZ" {
                    n208 = Variant To Data(type=w407, Variant=w410) -> (data=w406:dbl)  [unwired: 1 in, 1 out]
                  }
                }
                n209 = call "virtual XYZ rotator.vi"("current pos X"=w375, "current pos Y"=w375, "current pos Z"=w375, "virtual X relative"=w371, "virtual Y relative"=w370, "virtual Z relative"=w369) -> ("new pos X"=w383:dbl, "new pos Y"=w382:dbl, "new pos Z"=w381:dbl)  [unwired: 7 in]
                n210 = Bundle(cluster=w380, "moveXabs"=w383, "moveYabs"=w382, "moveZabs"=w381) -> (w378:T3)
                n211 = Bundle(cluster=w380, "moveXabs"=w371, "moveYabs"=w370, "moveZabs"=w369) -> (w379:T3)
                n212 = call-poly "GFGpolyGet.vi"("Variable Name in"="enable virtual XYZ") -> ("Boolean"=w377:bool)  [unwired: 10 in]
                n213 = Not(x=w377) -> (.not. x?=w376:bool)
                n214 = Select(t=w379, s=w376, f=w378) -> (s? t:f=w372:T3)
                n215 = call "GFG_core.vi"("Variable Name in"="moveXYZabs", "Variant in"=w372, "Action"=enum16{"Init", "Set", "Get"}."Set") -> ()  [unwired: 10 in, 7 out]
              }
            }
          }
          frame "enable.virtual.XYZ", "posX", "posY", "posZ" {
            w429 = T4 5 items=["X-Y-Z", "X-Z-Y", "Y-X-Z", "Y-Z-X", "Z-X-Y", "Z-Y-X", "X-Y-X", "X-Z-X", "Y-X-Y", "Y-Z-Y", "Z-X-Z", "Z-Y-Z"] ("rotation order")
            w443 = enum16{"Init", "Set", "Get"}."Set" ("Action")
            n216 = case shown="\"False\", Default" w442 {
              tunnel: w441 -> [_ w451]
              tunnel: [w447 w449] -> w418
              frame "False", Default {
                n217 = call-poly "GFGpolyGet.vi"("Variable Name in"="enable virtual XYZ") -> ("Boolean"=w447:bool)  [unwired: 10 in]
              }
              frame "enable.virtual.XYZ" {
                n218 = Variant To Data(type=TRUE, Variant=w451) -> (data=w449:bool)  [unwired: 1 in, 1 out]
                n219 = case shown="True" w449 {
                  frame False {
                  }
                  frame True {
                    n220 = call "set virtual Z rotation values.vi"() -> ()  [unwired: 12 in]
                  }
                }
              }
            }
            n221 = call-poly "GFGpolyGet.vi"("Variable Name in"="rot.vert") -> ("Numeric"=w433:dbl)  [unwired: 9 in, 1 out]
            n222 = call-poly "GFGpolyGet.vi"("Variable Name in"="rot.horiz") -> ("Numeric"=w432:dbl)  [unwired: 9 in, 1 out]
            n223 = Negate(x=w433) -> (-x=w435:dbl)
            n224 = Negate(x=w432) -> (-x=w434:dbl)
            n225 = Bundle(w434, w435, "phi"=0.0) -> (w437:cluster{dbl, dbl, "phi":dbl})  [unwired: 1 in]
            n226 = Not(x=w418) -> (.not. x?=w417:bool)
            n227 = call-poly "GFGpolyGet.vi"("Variable Name in"="posX") -> ("Numeric"=w427:dbl)  [unwired: 9 in, 1 out]
            n228 = call-poly "GFGpolyGet.vi"("Variable Name in"="posY") -> ("Numeric"=w426:dbl)  [unwired: 9 in, 1 out]
            n229 = call-poly "GFGpolyGet.vi"("Variable Name in"="posZ") -> ("Numeric"=w425:dbl)  [unwired: 9 in, 1 out]
            n230 = Bundle("Numeric"=w427, "Numeric"=w426, "Numeric"=w425) -> (w415:T5)  [unwired: 1 in]
            n231 = expression code="(x/180.0)*pi" "degrees to radians"(w437) -> (w428:cluster{dbl, dbl, "phi":dbl})
            n232 = Unbundle(w415) -> ("Numeric"=w424:dbl, "Numeric"=w423:dbl, "Numeric"=w422:dbl)
            n233 = call-poly <vilib>:"3D Cartesian Coordinate Rotation (Euler).vi"("rotation order"=w429, "Euler Angles"=w428, "z"=w422, "y"=w423, "x"=w424) -> ("z out"=w419:dbl, "y out"=w420:dbl, "x out"=w421:dbl)  [unwired: 3 in, 1 out]
            n234 = Bundle("x out"=w421, "y out"=w420, "z out"=w419) -> (w416:cluster{"x out":dbl, "y out":dbl, "z out":dbl})  [unwired: 1 in]
            n235 = Select(t=w415, s=w417, f=w416) -> (s? t:f=w414:cluster{"x out":dbl, "y out":dbl, "z out":dbl})
            n236 = Unbundle(w414) -> ("x out"=w413:dbl, "y out"=w412:dbl, "z out"=w411:dbl)
            n237 = call "GFG_core.vi"("Variable Name in"="setX", "Variant in"=w413, "Action"=w443) -> ()  [unwired: 10 in, 7 out]
            n238 = call "GFG_core.vi"("Variable Name in"="setY", "Variant in"=w412, "Action"=w443) -> ()  [unwired: 10 in, 7 out]
            n239 = call "GFG_core.vi"("Variable Name in"="setZ", "Variant in"=w411, "Action"=w443) -> ()  [unwired: 10 in, 7 out]
          }
          frame "QUIT" {
            n240 = Variant To Data(type=FALSE ("NewVal"), Variant=w454) -> (data=w452:bool)  [unwired: 1 in, 1 out]
          }
          frame "set.stage.speed" {
            n241 = call-poly "GFGpolyGet.vi"("Variable Name in"=w458) -> ("output cluster"=w457:T2)  [unwired: 9 in, 1 out]
            n242 = Unbundle By Name(w457) -> ("BooleanRef"=w456:refnum<vi>)
            n243 = call "set stage speeds.vi"() -> ()  [unwired: 12 in]
            n244 = property class="Bool"(reference=w456, "Value"=FALSE) -> ()  [unwired: 1 in, 2 out]
          }
        }
      }
    }
  }
